vi "Valve1DI1DO.vi"() -> ()   [LabVIEW 2019]
uses:
  TypeDef/ValveState.ctl
panel:
  out "Counter":u32
  in  "Reset":bool
  out "Unsheduled close":bool
  out "Unsheduled open":bool
  out "State":T1
  in  "CMD":bool
  out "DO":bool
  in  "DI":bool
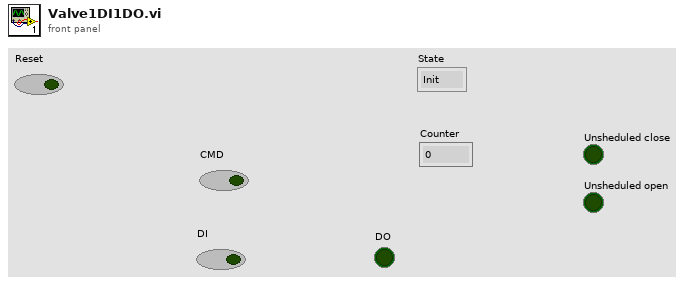
[diagram p1: front panel]
types:
  T1 = typedef "ValveState.ctl" = enum16{"Init", "Close", "Opening", "Open", "Closing"}
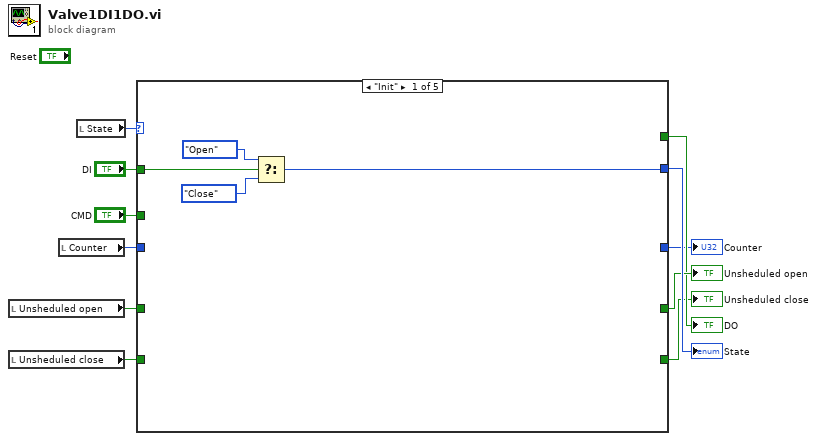
[diagram p0: block diagram]
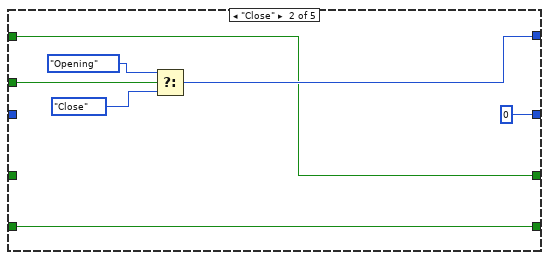
[diagram p2: hidden frame]
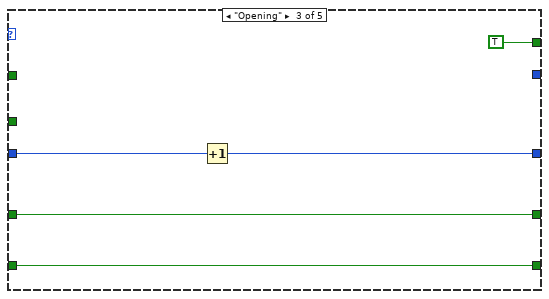
[diagram p3: hidden frame]
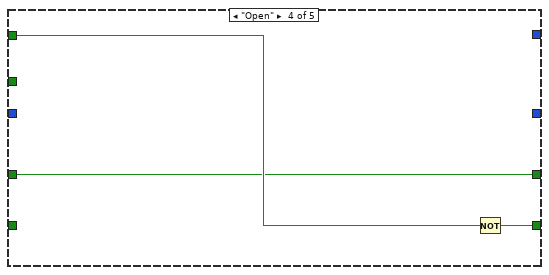
[diagram p4: hidden frame]
diagram:
  n1 = local read "Unsheduled open"() -> (w6:bool)
  n2 = local read "Unsheduled close"() -> (w3:bool)
  n3 = local read "Counter"() -> (w1:u32)
  n4 = local read "State"() -> (w11:T1)
  n5 = case shown="\"Init\"" w11 {
    tunnel: "DI" -> [w15 w18 _ w30 _]
    tunnel: [w12 w19 _ _ _] -> w9
    tunnel: "CMD" -> [_ w22 _ _ _]
    tunnel: [_ w18 w24 w28 _] -> w7
    tunnel: w6 -> [_ _ w24 w28 _]
    tunnel: [_ _ TRUE _ _] -> w5
    tunnel: [_ w17 w23 w29 _] -> w4
    tunnel: w3 -> [_ w17 w23 _ _]
    tunnel: [_ u32 0 w25 _ _] -> w2
    tunnel: w1 -> [_ _ w26 _ _]
    frame "Init" {
      n6 = Select(t=ValveState."Open" ("State"), s=w15, f=ValveState."Close" ("State")) -> (s? t:f=w12:T1)
    }
    frame "Close" {
      n7 = Select(t=ValveState."Opening" ("State"), s=w22, f=ValveState."Close" ("State")) -> (s? t:f=w19:T1)
    }
    frame "Opening" {
      n8 = Increment(x=w26) -> (x+1=w25:u32)
    }
    frame "Open" {
      n9 = Not(x=w30) -> (.not. x?=w29:bool)
    }
    frame "Closing" {
    }
  }
  "DO" <- w5
  "State" <- w9
  "Unsheduled open" <- w7
  "Unsheduled close" <- w4
  "Counter" <- w2
